vi "close_and_dereg_window.vi"(7 "error in":errorcluster, 10 "window":T1) -> (0 "error out":errorcluster)   [LabVIEW 2009]
uses:
  child window props.ctl
  FG states.ctl
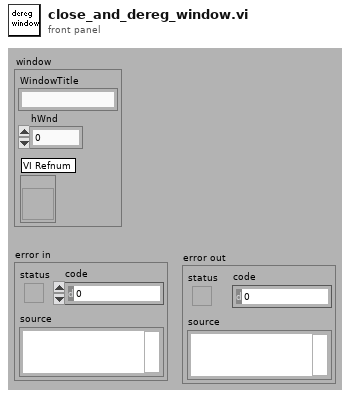
[diagram p1: front panel]
types:
  T1 = typedef "child window props.ctl" = cluster{"WindowTitle":string, "hWnd":u32, "VI Refnum":refnum<vi>}
  T2 = enum32{"Invalid", "Standard", "Closed", "Hidden", "Minimized", "Maximized"}
  T3 = typedef "FG states.ctl" = enum16{"init", "add", "replace", "remove", "read"}
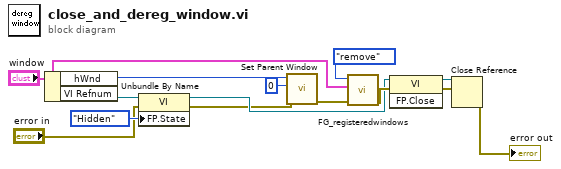
[diagram p0: block diagram]
diagram:
  n1 = Unbundle By Name("window") -> ("hWnd"=w9:u32, "VI Refnum"=w5:refnum<vi>)
  n2 = property class="VI"(reference=w5, error in="error in", "FP.State"=T2."Hidden" ("Front Panel Window:State")) -> (reference out=w3:refnum<vi>, error out=w1:errorcluster)
  n3 = call "Set Parent Window.vi"("error in (no error)"=w1, "new parent"=u16 0, "child"=w9) -> ("error out"=w7:errorcluster)  [unwired: 1 in, 7 out]
  n4 = call "FG_registeredwindows.vi"("error in (no error)"=w7, "window"="window", "action"=FG_states."remove") -> ("error out"=w14:errorcluster)  [unwired: 8 out]
  n5 = invoke class="VI" method="FP.Close"(reference=w3, error in=w14) -> (reference out=w11:refnum<vi>, error out=w12:errorcluster)  [unwired: 1 in, 1 out]
  n6 = Close Reference(reference=w11, error in (no error)=w12) -> (error out=→"error out":errorcluster)
